vi "OCR_Test_First_3_digit_13Aug21.vi"(0 "x":sgl=691.6022, 5 "Image File Path":path=path "C:/images/img1.jpeg", 7 "y":sgl=311.83267, 9 "Image in":T1(plugin-control)=refnum, 12 "error in (no error)":errorcluster) -> (3 "Read Top":string="6 G D", 6 "Read Center":string="6 G D" caption="Read String", 10 "Image":T1(plugin-control), 14 "Read bottom":string="D 6 D", 15 "error out":errorcluster)   [LabVIEW 2019]
uses:
  <vilib>/vision/NI_Vision_Development_Module.lvlib
panel:
  in  "Training File Path":path=path "D:/Focusing Station/Sub VIs/OCR_Test_18Aug21.abc"
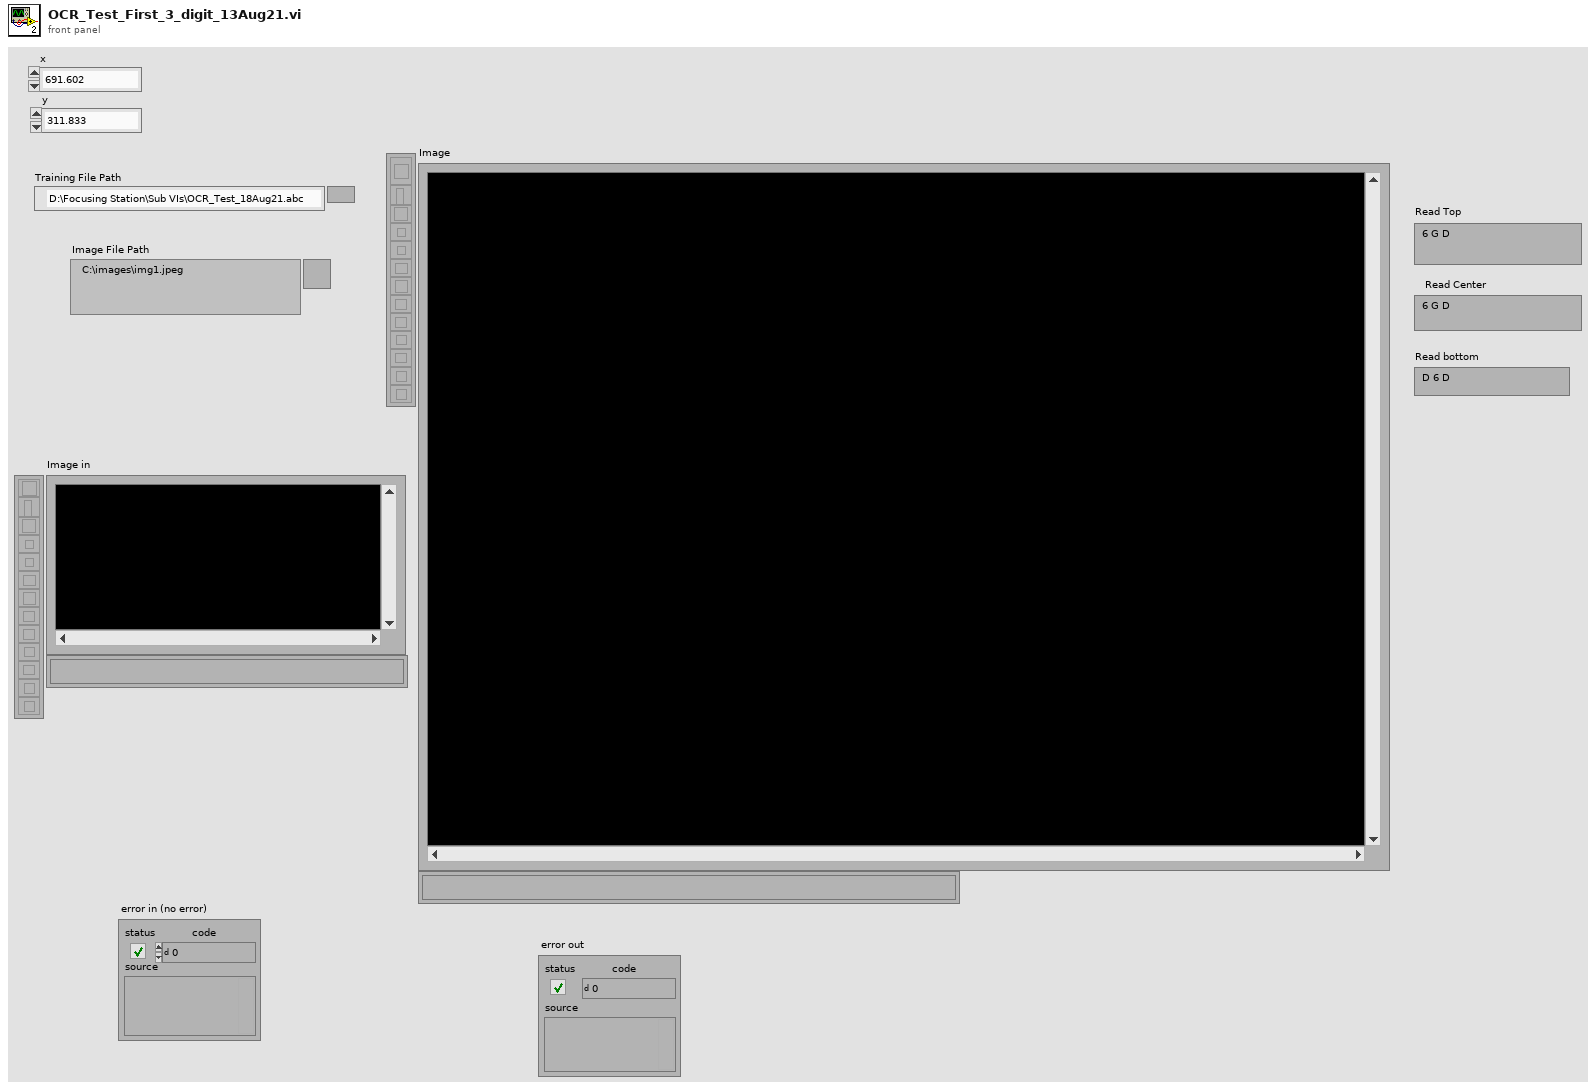
[diagram p1: front panel]
types:
  T1 = typedef "IMAQ Image.ctl" = refnum<image>
  T2 = typedef "IMAQ Rectangle" = cluster{"Left":i32, "Top":i32, "Right":i32, "Bottom":i32, "Rotation":dbl}
  T3 = typedef "Image Type" = u32
  T4 = typedef "IMAQ OCR Session.ctl" = refnum<k1>
  T5 = typedef "ROI Descriptor" = cluster{"Global Rectangle":i32[], "Contours":cluster{"ID":enum32{"External", "Internal"}, "Type":u32, "Coordinates":i32[]}[]}
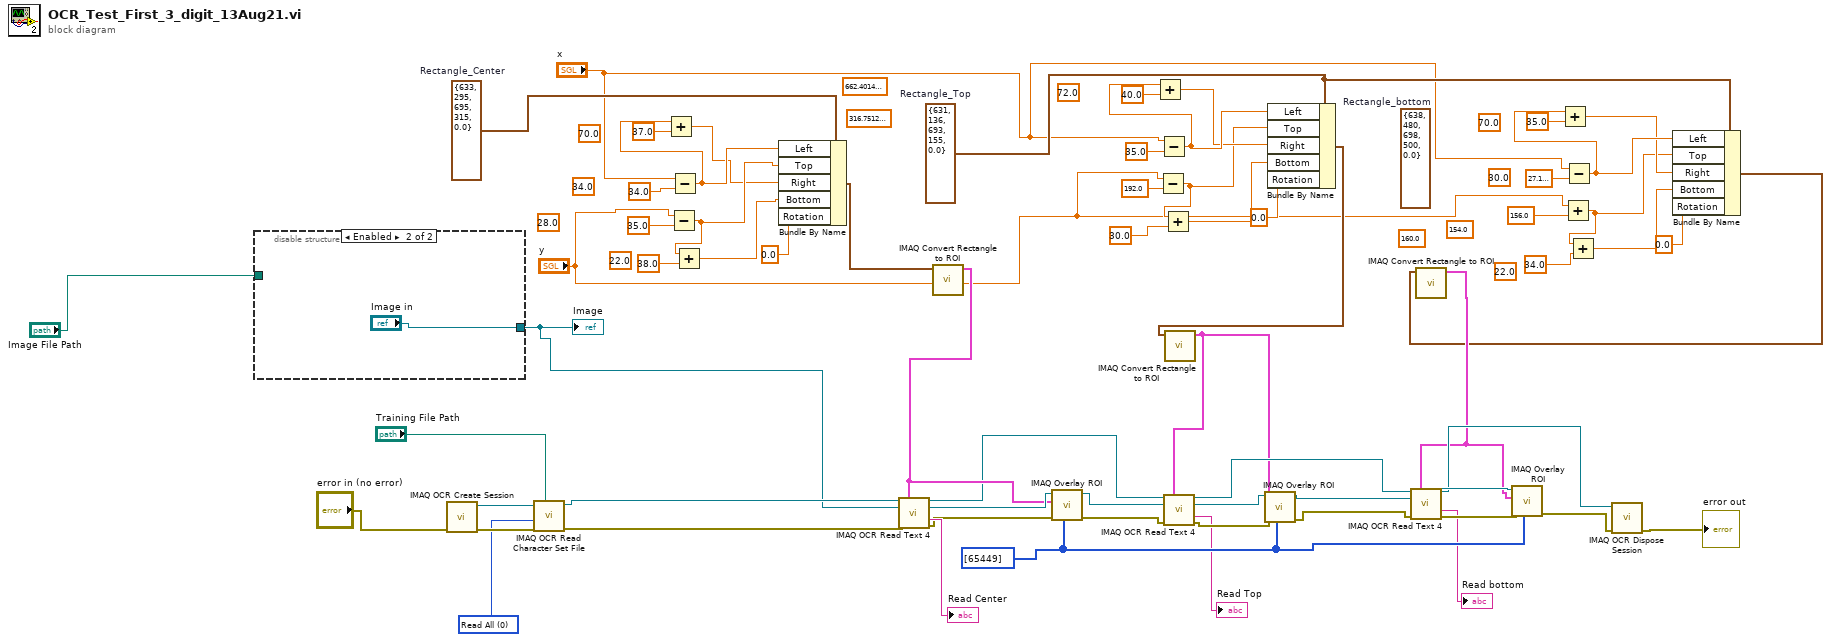
[diagram p0: block diagram]
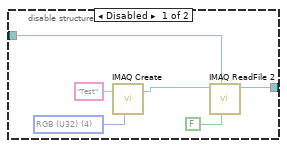
[diagram p2: hidden frame]
diagram:
  (unwired) sgl 30.0 ("y")
  (unwired) sgl 34.0 ("y")
  (unwired) sgl 70.0 ("y")
  (unwired) sgl 70.0 ("y")
  (unwired) sgl 72.0 ("y")
  (unwired) sgl 154.0 ("y")
  (unwired) sgl 22.0 ("y")
  (unwired) sgl 28.0 ("y")
  (unwired) sgl 22.0 ("y")
  (unwired) sgl 160.0 ("y")
  (unwired) sgl 316.75128 ("y")
  (unwired) sgl 662.4014 ("x")
  (unwired) T2 {"Left"=638, "Top"=480, "Right"=698, "Bottom"=500, "Rotation"=0.0}  # Rectangle_bottom
  w18 = T2 {"Left"=631, "Top"=136, "Right"=693, "Bottom"=155, "Rotation"=0.0}  # Rectangle_Top
  w56 = 0 items=["Read All", "Read Character Set Only", "Read Properties Only"] ("Read Options")
  w14 = T2 {"Left"=633, "Top"=295, "Right"=695, "Bottom"=315, "Rotation"=0.0}  # Rectangle_Center
  w40 = u32[] [65449] ("Colors (Green)")
  n1 = disable-structure shown="Enabled" {
    disable-tunnel: [w67 "Image in"] -> w60
    disable-tunnel: "Image File Path" -> [w66 _]
    frame Disabled {
      w68 = T3 4 items=["Grayscale (U8)", "Grayscale (I16)", "Grayscale (SGL)", "Complex (CSG)", "RGB (U32)", "HSL (U32)", "RGB (U64)", "Grayscale (U16)"] ("Image Type")
      n2 = call "IMAQ Create"("Image Name"="Test", "Image Type"=w68) -> ("New Image"=w70:T1)  [unwired: 3 in, 1 out]
      n3 = call "IMAQ ReadFile 2"("Use File Path Image Type"=FALSE, "File Path"=w66, "Image"=w70) -> ("Image Out"=w67:T1)  [unwired: 4 in, 4 out]
    }
    frame Enabled {
    }
  }
  "Image" <- w60
  n4 = call "IMAQ OCR Create Session"("error in (no error)"="error in (no error)") -> ("error out"=w64:errorcluster, "IMAQ OCR Session"=w65:T4)  [unwired: 9 in]
  n5 = call "IMAQ OCR Read Character Set File"("File Path"="Training File Path", "error in (no error)"=w64, "Read Options"=w56, "IMAQ OCR Session"=w65) -> ("error out"=w61:errorcluster, "IMAQ OCR Session (dup)"=w62:T4)  [unwired: 5 in, 1 out]
  n6 = Subtract(x="y", y=sgl 35.0) -> (x-y=w10:sgl)
  n7 = Subtract(x="x", y=sgl 34.0) -> (x-y=w11:sgl)
  n8 = Add(x=w11, y=sgl 37.0) -> (x+y=w9:sgl)
  n9 = Add(x=w10, y=sgl 38.0) -> (x+y=w8:sgl)
  n10 = Bundle By Name(cluster=w14, "Left"=w11, "Top"=w10, "Right"=w9, "Bottom"=w8, "Rotation"=0.0) -> (w7:T2)
  n11 = call "IMAQ Convert Rectangle to ROI"("Rectangle"=w7) -> ("ROI Descriptor"=w55:T5)  [unwired: 8 in, 1 out]
  n12 = call "IMAQ OCR Read Text 4"("IMAQ OCR Session"=w62, "ROI Descriptor"=w55, "Image"=w60, "error in (no error)"=w61) -> ("IMAQ OCR Session (dup)"=w50:T4, "Image (dup)"=w57:T1, "Read String"=→"Read Center":string, "error out"=w58:errorcluster)  [unwired: 5 in, 3 out]
  n13 = call "IMAQ Overlay ROI"("Colors (Green)"=w40, "error in (no error)"=w58, "ROI Descriptor"=w55, "Image"=w57) -> ("error out"=w48:errorcluster, "Image Out"=w49:T1)  [unwired: 2 in, 4 out]
  n14 = Subtract(x="y", y=sgl 192.0) -> (x-y=w28:sgl)
  n15 = Subtract(x="x", y=sgl 35.0) -> (x-y=w30:sgl)
  n16 = Add(x=w30, y=sgl 40.0) -> (x+y=w29:sgl)
  n17 = Add(x=w28, y=sgl 30.0) -> (x+y=w27:sgl)
  n18 = Bundle By Name(cluster=w18, "Left"=w30, "Top"=w28, "Right"=w29, "Bottom"=w27, "Rotation"=0.0) -> (w26:T2)
  n19 = call "IMAQ Convert Rectangle to ROI"("Rectangle"=w26) -> ("ROI Descriptor"=w36:T5)  [unwired: 8 in, 1 out]
  n20 = call "IMAQ OCR Read Text 4"("IMAQ OCR Session"=w50, "ROI Descriptor"=w36, "Image"=w49, "error in (no error)"=w48) -> ("IMAQ OCR Session (dup)"=w43:T4, "Image (dup)"=w52:T1, "Read String"=→"Read Top":string, "error out"=w51:errorcluster)  [unwired: 5 in, 3 out]
  n21 = call "IMAQ Overlay ROI"("Colors (Green)"=w40, "error in (no error)"=w51, "ROI Descriptor"=w36, "Image"=w52) -> ("error out"=w44:errorcluster, "Image Out"=w45:T1)  [unwired: 2 in, 4 out]
  n22 = Add(x="y", y=sgl 156.0) -> (x+y=w20:sgl)
  n23 = Subtract(x="x", y=sgl 27.1) -> (x-y=w22:sgl)
  n24 = Add(x=w22, y=sgl 35.0) -> (x+y=w21:sgl)
  n25 = Add(x=w20, y=sgl 34.0) -> (x+y=w19:sgl)
  n26 = Bundle By Name(cluster=w18, "Left"=w22, "Top"=w20, "Right"=w21, "Bottom"=w19, "Rotation"=0.0) -> (w17:T2)
  n27 = call "IMAQ Convert Rectangle to ROI"("Rectangle"=w17) -> ("ROI Descriptor"=w39:T5)  [unwired: 8 in, 1 out]
  n28 = call "IMAQ OCR Read Text 4"("IMAQ OCR Session"=w43, "ROI Descriptor"=w39, "Image"=w45, "error in (no error)"=w44) -> ("IMAQ OCR Session (dup)"=w42:T4, "Image (dup)"=w46:T1, "Read String"=→"Read bottom":string, "error out"=w47:errorcluster)  [unwired: 5 in, 3 out]
  n29 = call "IMAQ Overlay ROI"("Colors (Green)"=w40, "error in (no error)"=w47, "ROI Descriptor"=w39, "Image"=w46) -> ("error out"=w41:errorcluster)  [unwired: 2 in, 5 out]
  n30 = call "IMAQ OCR Dispose Session"("error in (no error)"=w41, "IMAQ OCR Session"=w42) -> ("error out"=→"error out":errorcluster)  [unwired: 9 in]
